vi "OQCN_LaunchPad.vi"() -> ()   [LabVIEW 2015]
uses:
  <vilib>/Analysis/NI_AALBase.lvlib
panel:
  out "trigger flag":bool
  in  "stop 2":bool
  out "z var":dbl format="%0.2f"
  out "y var":dbl format="%0.2f"
  out "x var":dbl format="%0.2f"
  out "z st.d":dbl format="%0.2f"
  out "y st.d":dbl format="%0.2f"
  out "x st.d":dbl format="%0.2f"
  out "z mean":dbl format="%0.2f"
  in  "®z¾_                    «ØÄ³­È                                       ±j¾_":dbl(slide)=3.0229007633587788 scale=0.0..9.0 scale format="%#_1g"
  out "y mean":dbl format="%0.2f"
  out "x mean":dbl format="%0.2f"
  out "z":dbl
  out "y":dbl
  out "x":dbl
  out "trigger":bool
  out "init loop":i32
  in  "stop":bool
  out "CurrentPath":path=path "C:/Documents and Settings/TGI0362/My Documents/xUserData/LabVIEW_8.x/cmDVT_Factory-BBU-R5"
  out "new picture":picture
  # "OQCN LaunchPad\n°»´ú¾_°Ê"
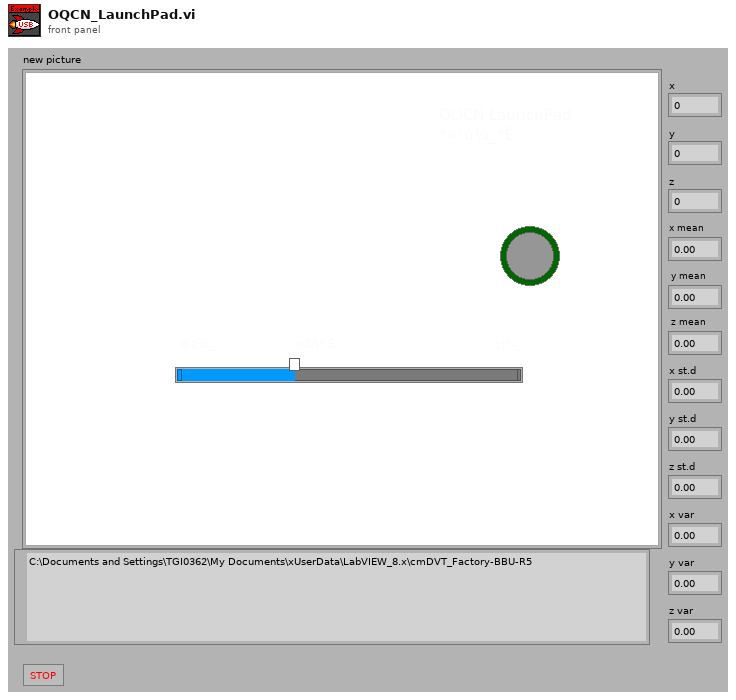
[diagram p1: front panel]
types:
  T1 = typedef "imagedata.ctl" = cluster{"image type":i32, "image depth":i32, "image":u8[], "mask":u8[], "colors":u32[], "Rectangle":cluster{"left":i16, "top":i16, "right":i16, "bottom":i16}}
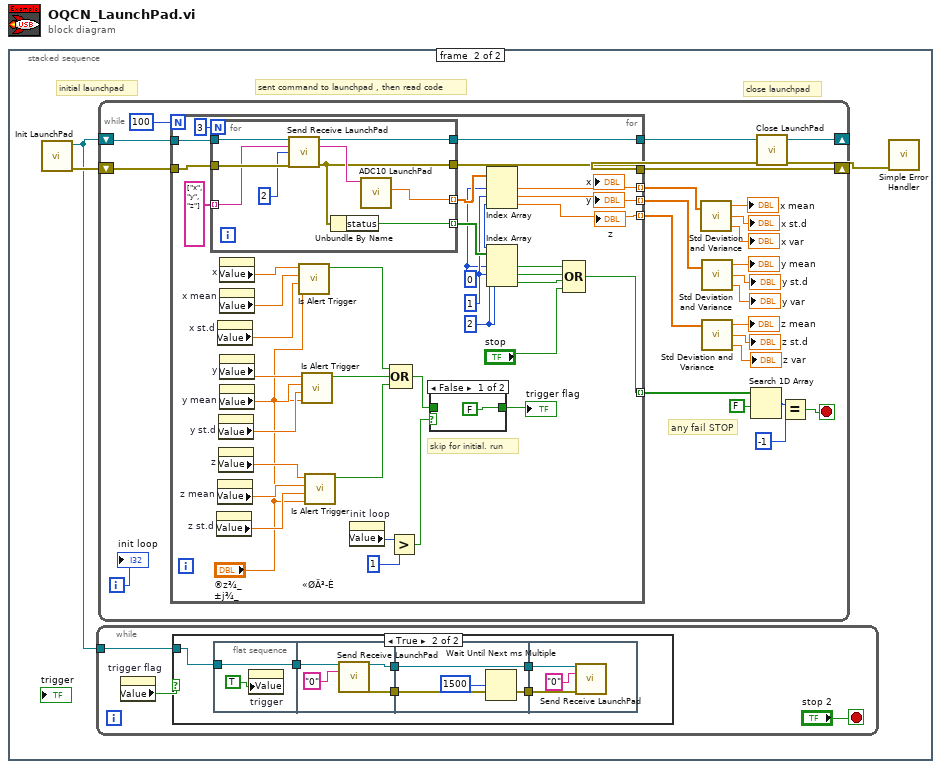
[diagram p0: block diagram]
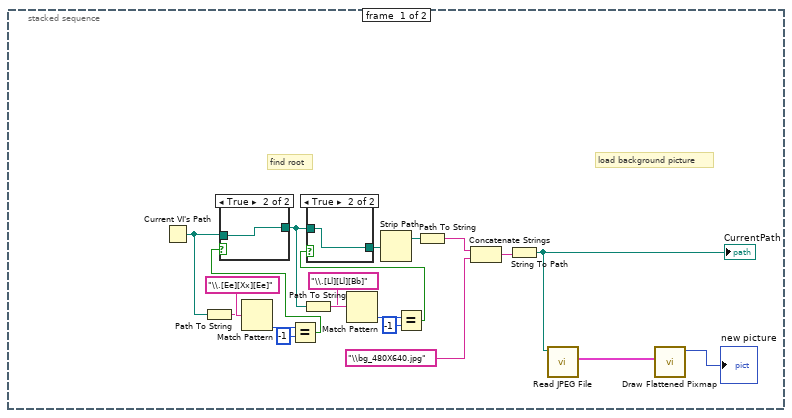
[diagram p2: hidden frame]
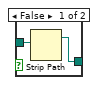
[diagram p3: hidden frame]
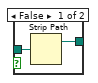
[diagram p4: hidden frame]
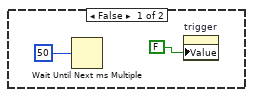
[diagram p5: hidden frame]
diagram:
  n1 = stacked-sequence {
    frame #0 {
      # "load background picture"
      # "find root"
      n2 = Current VI's Path() -> (path=w9:path)
      n3 = Path To String(path=w9) -> (string=w8:string)
      n4 = Match Pattern(string=w8, regular expression="\\.[Ee][Xx][Ee]") -> (offset past match=w6:i32)  [unwired: 1 in, 3 out]
      n5 = Equal?(x=w6, y=-1) -> (x = y?=w18:bool)
      n6 = case shown="True" w18 {
        tunnel: [w24 w26] -> w15
        tunnel: w9 -> [w25 w26]
        frame False {
          n7 = Strip Path(path=w25) -> (stripped path=w24:path)  [unwired: 1 out]
        }
        frame True {
        }
      }
      n8 = Path To String(path=w15) -> (string=w12:string)
      n9 = Match Pattern(string=w12, regular expression="\\.[Ll][Ll][Bb]") -> (offset past match=w14:i32)  [unwired: 1 in, 3 out]
      n10 = Equal?(x=w14, y=-1) -> (x = y?=w17:bool)
      n11 = case shown="True" w17 {
        tunnel: [w21 w23] -> w16
        tunnel: w15 -> [w22 w23]
        frame False {
          n12 = Strip Path(path=w22) -> (stripped path=w21:path)  [unwired: 1 out]
        }
        frame True {
        }
      }
      n13 = Strip Path(path=w16) -> (stripped path=w5:path)  [unwired: 1 out]
      n14 = Path To String(path=w5) -> (string=w2:string)
      n15 = Concatenate Strings(w2, "\\bg_480X640.jpg") -> (w3:string)
      n16 = String To Path(string=w3) -> (path=w1:path)
      "CurrentPath" <- w1
      n17 = call <vilib>:"Read JPEG File.vi"("path to JPEG file"=w1) -> ("image data"=w19:T1)  [unwired: 8 in, 2 out]
      n18 = call <vilib>:"Draw Flattened Pixmap.vi"("image data"=w19) -> ("new picture"=→"new picture":picture)  [unwired: 8 in]
    }
    frame #1 {
      # "close launchpad"
      # "sent command to launchpad , then read code"
      # "initial launchpad"
      n19 = call "Init LaunchPad.vi"() -> ("error out"=w29:errorcluster, "VISA resource name out"=w27:refnum<visa-resource-name>)  [unwired: 10 in]
      n20 = while {
        tunnel: w27 -> [w32]
        stop <- "stop 2" stop-if-true
        n21 = property on="trigger flag" class="Bool (strict)"() -> ("Value"=w33:bool)  [unwired: 2 in, 2 out]
        n22 = case shown="True" w33 {
          tunnel: w32 -> [_ w42]
          frame False {
            n23 = Wait Until Next ms Multiple(millisecond multiple=u32 50) -> ()  [unwired: 1 out]
            n24 = property on="trigger" class="Bool (strict)"("Value"=FALSE) -> ()  [unwired: 2 in, 2 out]
          }
          frame True {
            n25 = flat-sequence {
              tunnel: w42 -> [w44]
              tunnel: [w44] -> w37
              tunnel: [w46] -> w41
              tunnel: [w45] -> w39
              tunnel: w37 -> [w48]
              tunnel: w41 -> [w50]
              tunnel: [w50] -> w40
              tunnel: w39 -> [w49]
              tunnel: [w49] -> w38
              tunnel: w40 -> [w53]
              tunnel: w38 -> [w52]
              frame #0 {
                n26 = property on="trigger" class="Bool (strict)"("Value"=TRUE) -> ()  [unwired: 2 in, 2 out]
              }
              frame #1 {
                n27 = call "Send Receive LaunchPad.vi"("VISA resource"=w48, "write buffer"="0") -> ("VISA resource 2"=w46:refnum<visa-resource-name>, "error out"=w45:errorcluster)  [unwired: 11 in, 1 out]
              }
              frame #2 {
                n28 = Wait Until Next ms Multiple(millisecond multiple=u32 1500) -> ()  [unwired: 1 out]
              }
              frame #3 {
                n29 = call "Send Receive LaunchPad.vi"("VISA resource"=w53, "write buffer"="0", "error in"=w52) -> ()  [unwired: 10 in, 3 out]
              }
            }
          }
        }
      }
      n30 = while {
        shift-right: [w77] -> w30
        shift-left: w29 -> [w76]
        shift-right: [w75] -> w28
        shift-left: w27 -> [w74]
        i -> [w55]
        stop <- w68 stop-if-true
        # "any fail STOP"
        n31 = for {
          N: 100 -> [_]
          tunnel: [w107] -> w60 mode=indexing
          tunnel: [w106] -> w77
          tunnel: w76 -> [w105]
          tunnel: [w104] -> w75
          tunnel: w74 -> [w103]
          tunnel: [w98] -> w72 mode=indexing
          tunnel: [w97] -> w61 mode=indexing
          tunnel: [w96] -> w56 mode=indexing
          w101 = 2 ("index")
          w100 = 1 ("index")
          w99 = 0 ("index")
          # "skip for initial. run"
          n32 = for {
            N: 3 -> [_]
            tunnel: w103 -> [w125]
            tunnel: [w124] -> w104
            tunnel: [w118] -> w106
            tunnel: w105 -> [w123]
            tunnel: string[] ["x", "y", "z"] -> [w121] mode=indexing
            tunnel: [w119] -> w102 mode=indexing
            tunnel: [w117] -> w112 mode=indexing
            n33 = call "Send Receive LaunchPad.vi"("VISA resource"=w125, "write buffer"=w121, "Bytes To Read (0)"=u8 2, "error in"=w123) -> ("VISA resource 2"=w124:refnum<visa-resource-name>, "Read Buffer"=w120:string, "error out"=w118:errorcluster)  [unwired: 9 in]
            n34 = Unbundle By Name(w118) -> ("status"=w117:bool)
            n35 = call "ADC10 LaunchPad.vi"("string"=w120) -> ("ADC10 (Volt)"=w119:dbl)  [unwired: 9 in, 1 out]
          }
          n36 = property on="z st.d" class="DigNum (strict)"() -> ("Value"=w87:dbl)  [unwired: 2 in, 2 out]
          n37 = property on="x st.d" class="DigNum (strict)"() -> ("Value"=w93:dbl)  [unwired: 2 in, 2 out]
          n38 = property on="z mean" class="DigNum (strict)"() -> ("Value"=w88:dbl)  [unwired: 2 in, 2 out]
          n39 = property on="y st.d" class="DigNum (strict)"() -> ("Value"=w90:dbl)  [unwired: 2 in, 2 out]
          n40 = property on="z" class="DigNum (strict)"() -> ("Value"=w89:dbl)  [unwired: 2 in, 2 out]
          n41 = property on="x" class="DigNum (strict)"() -> ("Value"=w95:dbl)  [unwired: 2 in, 2 out]
          n42 = property on="x mean" class="DigNum (strict)"() -> ("Value"=w94:dbl)  [unwired: 2 in, 2 out]
          n43 = property on="y" class="DigNum (strict)"() -> ("Value"=w92:dbl)  [unwired: 2 in, 2 out]
          n44 = property on="y mean" class="DigNum (strict)"() -> ("Value"=w91:dbl)  [unwired: 2 in, 2 out]
          n45 = call "Is Alert Trigger.vi"("times"="®z¾_                    «ØÄ³­È                                       ±j¾_", "standard deviation"=w93, "mean"=w94, "value"=w95) -> ("is alert?"=w85:bool)  [unwired: 7 in]
          n46 = call "Is Alert Trigger.vi"("times"="®z¾_                    «ØÄ³­È                                       ±j¾_", "standard deviation"=w90, "mean"=w91, "value"=w92) -> ("is alert?"=w84:bool)  [unwired: 7 in]
          n47 = call "Is Alert Trigger.vi"("times"="®z¾_                    «ØÄ³­È                                       ±j¾_", "standard deviation"=w87, "mean"=w88, "value"=w89) -> ("is alert?"=w83:bool)  [unwired: 7 in]
          n48 = property on="init loop" class="DigNum (strict)"() -> ("Value"=w82:i32)  [unwired: 2 in, 2 out]
          n49 = Greater?(x=w82, y=1) -> (0:w80:bool)
          n50 = Compound Arithmetic op=OR(w85, w84, w83) -> (w79:bool)
          n51 = case shown="False" w80 {
            tunnel: w79 -> [_ w116]
            tunnel: [FALSE ("element") w116] -> w78
            frame False {
            }
            frame True {
            }
          }
          "trigger flag" <- w78
          n52 = Index Array(array=w102, index #1=w99, index #2=w100, index #3=w101) -> (element #1=w98:dbl, element #2=w97:dbl, element #3=w96:dbl)
          "x" <- w98
          "y" <- w97
          "z" <- w96
          n53 = Index Array(array=w112, index #1=w99, index #2=w100, index #3=w101) -> (element #1=w111:bool, element #2=w110:bool, element #3=w109:bool)
          n54 = Compound Arithmetic op=OR(w111, w110, w109, "stop") -> (w107:bool)
        }
        n55 = call <vilib>:"Std Deviation and Variance.vi"("X"=w72) -> ("mean"=→"x mean":dbl, "standard deviation"=→"x st.d":dbl, "variance"=→"x var":dbl)  [unwired: 1 in]
        n56 = call <vilib>:"Std Deviation and Variance.vi"("X"=w61) -> ("mean"=→"y mean":dbl, "standard deviation"=→"y st.d":dbl, "variance"=→"y var":dbl)  [unwired: 1 in]
        n57 = call <vilib>:"Std Deviation and Variance.vi"("X"=w56) -> ("mean"=→"z mean":dbl, "standard deviation"=→"z st.d":dbl, "variance"=→"z var":dbl)  [unwired: 1 in]
        n58 = Search 1D Array(1D array=w60, element=FALSE) -> (index of element=w71:i32)  [unwired: 1 in]
        n59 = Equal?(x=w71, y=-1) -> (x = y?=w68:bool)
        "init loop" <- w55
      }
      n60 = call "Close LaunchPad.vi"("VISA resource name"=w28, "error in"=w30) -> ("error out"=w31:errorcluster)  [unwired: 13 in]
      n61 = call <vilib>:"Simple Error Handler.vi"("error in (no error)"=w31) -> ()  [unwired: 4 in, 5 out]
    }
  }
